vi "[GlobVar]Param.vi"() -> ()   [LabVIEW 2018]
panel:
  in  "PumpPressureThreshold":dbl format="%#_g bar"
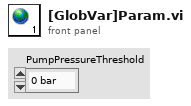
[diagram p1: front panel]
diagram:
